vi "Set Output Mode.vi"(8 "error in (no error)":errorcluster caption="错误输入（无错误）", 10 "Output Mode":u32(ring) items=["Standby", "Operate"], 11 "Simulation Source 输入":refnum<class "Simulation Source.lvclass">) -> (0 "error out":errorcluster caption="错误输出", 3 "Simulation Source 输出":refnum<class "Simulation Source.lvclass">)   [LabVIEW 2020, in "Simulation Source.lvlib" / "Simulation Source.lvclass"]
uses:
  Simulation Source.lvclass
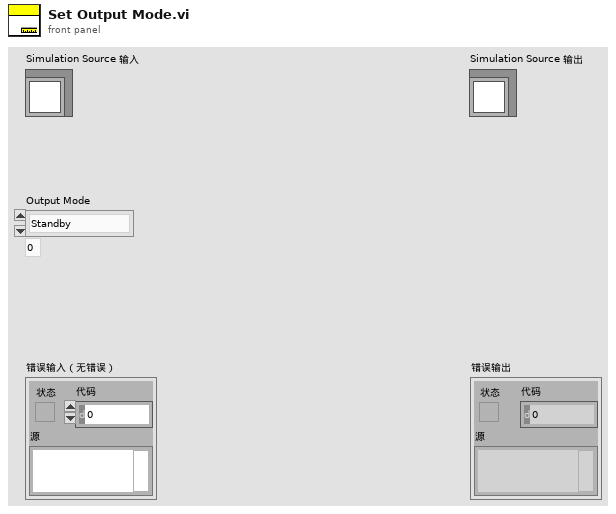
[diagram p1: front panel]
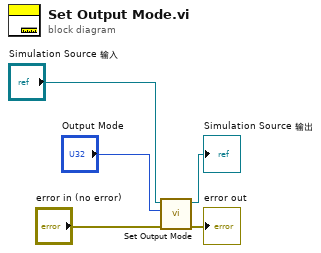
[diagram p0: block diagram]
diagram:
  n1 = call-parent "Set Output Mode.vi"("error in (no error)"="error in (no error)", "Output Mode"="Output Mode", "多功能校准源接口 输入"="Simulation Source 输入") -> ("error out"=→"error out":errorcluster, "多功能校准源接口 输出"=→"Simulation Source 输出":refnum<class "Simulation Source.lvclass">)  [unwired: 7 in]
